vi "Update Builds.vi"(8 "error in (no error)":errorcluster, 10 "Builds":T1[](array[typedef]), 11 "GVIWebProcessorApp in":refnum<class "GVIWebProcessorApp.lvclass">) -> (0 "error out":errorcluster, 3 "GVIWebProcessorApp out":refnum<class "GVIWebProcessorApp.lvclass">)   [LabVIEW 2020, in "PicoG-Processor.lvlib" / "GVIWebProcessorApp.lvclass"]
uses:
  GVIWebProcessorApp.lvclass
  WebProjectPanel/WebProjectPanel.lvclass
  <vilib>/IlluminatedG/IG OOPanel/OOPanel/ArrayManager/ArrayManager.lvclass
  PicoG-Processor.lvlib
  <vilib>/IlluminatedG/IG OOPanel/OOPanel/Panel/Panel.lvclass
  C:/Program Files (x86)/National Instruments/LabVIEW 2020/vi.lib/IlluminatedG/IG OOPanel/OOPanel/ArrayPanel/ArrayPanel.lvclass
  C:/Program Files (x86)/National Instruments/LabVIEW 2020/vi.lib/IlluminatedG/IG OOPanel/OOPanel/Panel/Panel.lvclass
  C:/dev/Vireo/PicoG/PicoG-Processor/WebProjectPanel/WebProjectPanel.lvclass
  WebProjectWatcher/Web Build.ctl
  WebProjectWatcher/WebProjectWatcher.lvclass
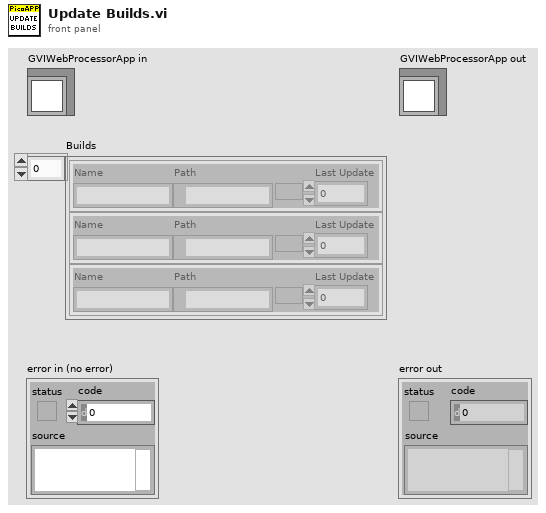
[diagram p1: front panel]
types:
  T1 = typedef "PicoG-Processor.lvlib/WebProjectWatcher.lvclass/Web Build.ctl" = cluster{"Name":string, "Path":path, "Last Update":dbl}
  T2 = map{path, refnum<class "WebProjectPanel.lvclass">}
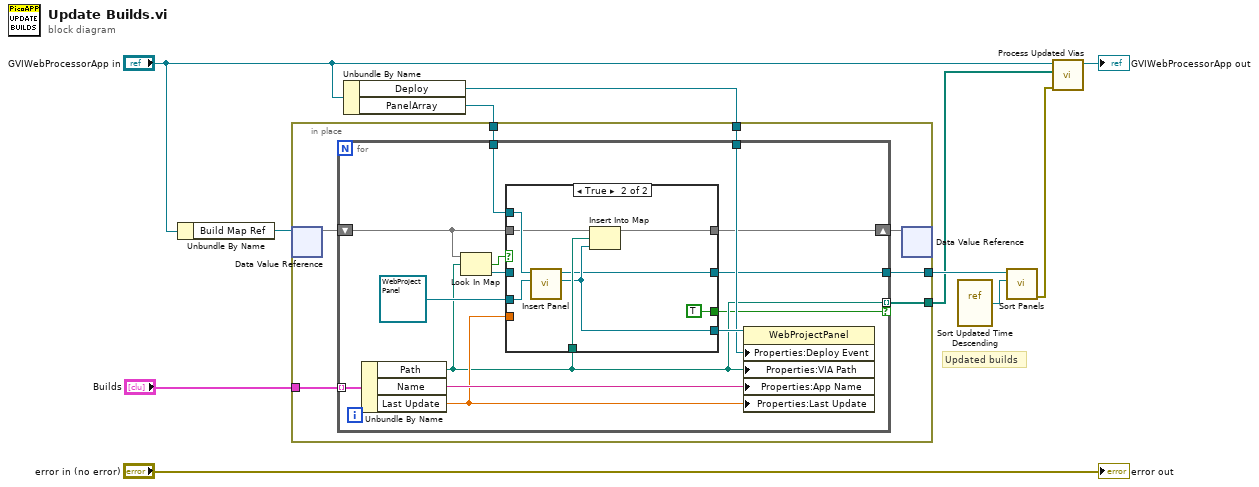
[diagram p0: block diagram]
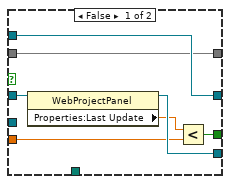
[diagram p2: hidden frame]
diagram:
  # "Updated builds"
  n1 = Unbundle By Name("GVIWebProcessorApp in") -> ("Build Map Ref"=w5:refnum<data-value>)
  n2 = Unbundle By Name("GVIWebProcessorApp in") -> ("Deploy"=w9:refnum<user-event>, "PanelArray"=w10:refnum<class "ArrayManager.lvclass">)
  n3 = in-place {
    in-place-border: w10 -> [w18]
    in-place-border: w9 -> [w17]
    in-place-border: [w16] -> w8
    in-place-border: "Builds" -> [w15]
    in-place-border: [w12] -> w1
    n4 = in-place-dvr #1(w5) -> (w14:T2)  [unwired: 1 out]
    n5 = for {
      tunnel: w15 -> [w32] mode=indexing
      tunnel: w18 -> [w30]
      tunnel: w17 -> [w26]
      tunnel: [w24] -> w16
      tunnel: [w22] -> w12 mode=indexing if=w21
      shift-right: [w19] -> w13
      shift-left: w14 -> [w20]
      n6 = Unbundle By Name(w32) -> ("Path"=w22:path, "Name"=w27:string, "Last Update"=w23:dbl)
      n7 = Look In Map(map=w20, key=w22) -> (key not found?=w31:bool, value=w29:refnum<class "WebProjectPanel.lvclass">)  [unwired: 1 in]
      n8 = case shown="True" w31 {
        tunnel: w22 -> [_ w45]
        tunnel: w30 -> [w39 w47]
        tunnel: w29 -> [w38 _]
        tunnel: w20 -> [w33 w46]
        tunnel: [w37 w44] -> w28
        tunnel: refnum<class "WebProjectPanel.lvclass"> refnum ("PicoG-Processor:WebProjectPanel.lvclass") -> [_ w43]
        tunnel: [w39 w42] -> w24
        tunnel: w23 -> [w35 _]
        tunnel: [w34 TRUE] -> w21
        tunnel: [w33 w40] -> w19
        frame False {
          n9 = property class="WebProjectPanel"(reference=w38) -> (reference out=w37:refnum<class "WebProjectPanel.lvclass">, "Properties:Last Update"=w36:dbl)  [unwired: 1 in, 1 out]
          n10 = Less?(x=w36, y=w35) -> (x < y?=w34:bool)
        }
        frame True {
          n11 = call <vilib>:"Insert Panel.vi"("Panel/Type"=w43, "PanelArray in"=w47) -> ("Panel"=w44:refnum<class "WebProjectPanel.lvclass">, "PanelArray out"=w42:refnum<class "ArrayManager.lvclass">)  [unwired: 7 in, 1 out]
          n12 = Insert Into Map(map in=w46, key=w45, value=w44) -> (map out=w40:T2)  [unwired: 2 out]
        }
      }
      n13 = property class="WebProjectPanel"(reference=w28, "Properties:Deploy Event"=w26, "Properties:VIA Path"=w22, "Properties:App Name"=w27, "Properties:Last Update"=w23) -> ()  [unwired: 1 in, 2 out]
    }
    n14 = in-place-dvr #1(w13) -> ()  [unwired: 2 out]
  }
  n15 = vi-ref "Sort Updated Time Descending.vi"() -> (w7:refnum<vi>)
  n16 = call <vilib>:"Sort Panels.vi"("Sort VI"=w7, "ArrayManager in"=w8) -> ("error out"=w3:errorcluster)  [unwired: 8 in, 1 out]
  n17 = call "Process Updated Vias.vi"("error in (no error)"=w3, "Via Paths"=w1, "GVIWebProcessorApp in"="GVIWebProcessorApp in") -> ("GVIWebProcessorApp out"=→"GVIWebProcessorApp out":refnum<class "GVIWebProcessorApp.lvclass">)  [unwired: 7 in, 1 out]
  "error out" <- "error in (no error)"
